vi "WaitforServerToStart.vi"(1 "ROS in":T1) -> (0 "ROS out":T1)   [LabVIEW 2015]
uses:
  _ROSControl.ctl
  _ROSDirection.ctl
  Console/Servers/ServerSubs/MyState.ctl
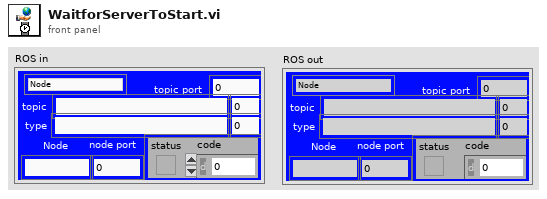
[diagram p1: front panel]
types:
  T1 = typedef "_ROSControl.ctl" = cluster{"topic port":u16, "Node":string, "topic":string, "type":string, "node port":u16, "error ":errorcluster, "Direction":T2, "Update (ms)":u16, "FIFO size":u16}
  T2 = typedef "_ROSDirection.ctl" = enum16{"Node", "Publisher", "Subscriber", "ServiceClient", "ServiceProvider"}
  T3 = typedef "MyState.ctl" = enum16{"No Connection", "Registered", "Connected", "Close"}
  T4 = typedef "ServoInfo.ctl" = cluster{"vi name":string, "queue":refnum<queue>, "ROS":T1, "notifier":refnum<notifier>, "FIFO":refnum<queue>, "This VI":refnum<vi>, "MyState":T3}
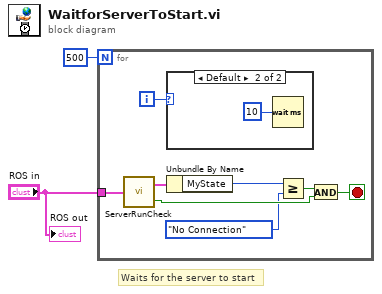
[diagram p0: block diagram]
diagram:
  # "Waits for the server to start"
  n1 = for {
    N: 500 -> [_]
    tunnel: "ROS in" -> [w10]
    i -> [w5]
    stop <- w6 stop-if-true
    n2 = call "ServerRunCheck.vi"("ROS in"=w10) -> ("Running?"=w7:bool, "ServerFound"=w9:T4)
    n3 = case shown="Default" w5 {
      frame 0 {
      }
      frame Default {
        n4 = Wait (ms)(milliseconds to wait=u32 10) -> ()  [unwired: 1 out]
      }
    }
    n5 = Unbundle By Name(w9) -> ("MyState"=w4:T3)
    n6 = Greater Or Equal?(x=w4, y=MyState."No Connection" ("x")) -> (x >= y?=w8:bool)
    n7 = And(x=w8, y=w7) -> (x .and. y?=w6:bool)
  }
  "ROS out" <- "ROS in"
